vi "VideoRecorderMini.vi"() -> ()   [LabVIEW 2010]
uses:
  <instrlib>/niHWS/nihws.llb/niHWS Open File Permissions ID.ctl
  <vilib>/DAQmx/read.llb/DAQmx Read (Analog 1D Wfm NChan NSamp).vi
  <vilib>/DAQmx/create/channels.llb/DAQmx Create Channel (AI-Voltage-Basic).vi
  <vilib>/DAQmx/configure/timing.llb/DAQmx Timing (Sample Clock).vi
  <vilib>/daqmx/miscellaneous.llb/DAQmx Fill In Error Info.vi
  <instrlib>/niHWS/nihws.llb/niHWS Write Analog WDT.vi
  <instrlib>/niHWS/nihws.llb/niHWS Write Analog DBL.vi
  <vilib>/vision/driver/NI_Vision_Acquisition_Software.lvlib
  C:/Program Files/National Instruments/LabVIEW 2010/resource/objmgr/imaqdx.rc
  <vilib>/ptbypt/NI_PtbyPt.lvlib
  C:/Program Files/National Instruments/LabVIEW 2010/resource/objmgr/daqmx.rc
  <vilib>/vision/NI_Vision_Development_Module.lvlib
panel:
  in  "Ephys":bool=TRUE
  in  "Video":bool=TRUE
  in  "Downsampling factor":i32=15
  in  "reduce size":bool
  in  "Channel Names":string[](array[string])
  out "Ephys Recoding Signals":waveform(dbl)[](graph)
  in  "Recording channels":tag="PXI1Slot2/ai2"
  in  "Extra":bool=TRUE
  in  "Camera":string(combo)
  in  "Video Modes":string(combo)
  in  "Compressor":string(combo)
  in  "Selected Path for AVI":path
  in  "Rec":bool
  out "fps":dbl format="%#_2g"
  in  "% Quality":i32=-1
  in  "Start":bool
  in  "Display":bool
  out "Rec Time":dbl format="%#_3g"
  in  "stop":bool
  out "Image Out":T1(plugin-control)
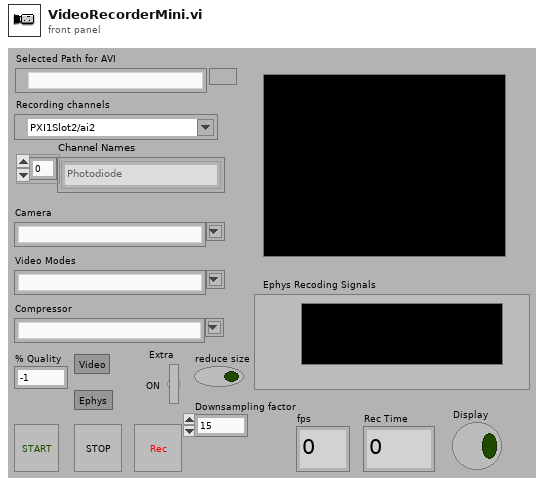
[diagram p1: front panel]
types:
  T1 = typedef "IMAQ Image.ctl" = refnum<image>
  T2 = typedef "niHWS Open File Permissions ID.ctl" = enum32{"Read Only", "Read/Write Existing", "Read/Write/Create New", "Read/Write/Create New Always"}
  T3 = cluster{"Type":u32, "Version":u32, "Flags":u32, "SerialNumberHigh":u32, "SerialNumberLow":u32, "BusType":u32, "InterfaceName":string, "VendorName":string, "ModelName":string, "CameraFileName":string, "CameraAttributeURL":string}[]
  T4 = cluster{"Type":u32, "Version":u32, "Flags":u32, "SerialNumberHigh":u32, "SerialNumberLow":u32, "BusType":u32, "InterfaceName":string, "VendorName":string, "ModelName":string, "CameraFileName":string, "CameraAttributeURL":string}
  T5 = typedef "IMAQdx.ctl" = refnum<k21>
  T6 = cluster{"Video Mode":u32, "Video Mode Name":string}[]
  T7 = typedef "AviRefnum.ctl" = refnum<k1>
  T8 = typedef "Image Type" = u32
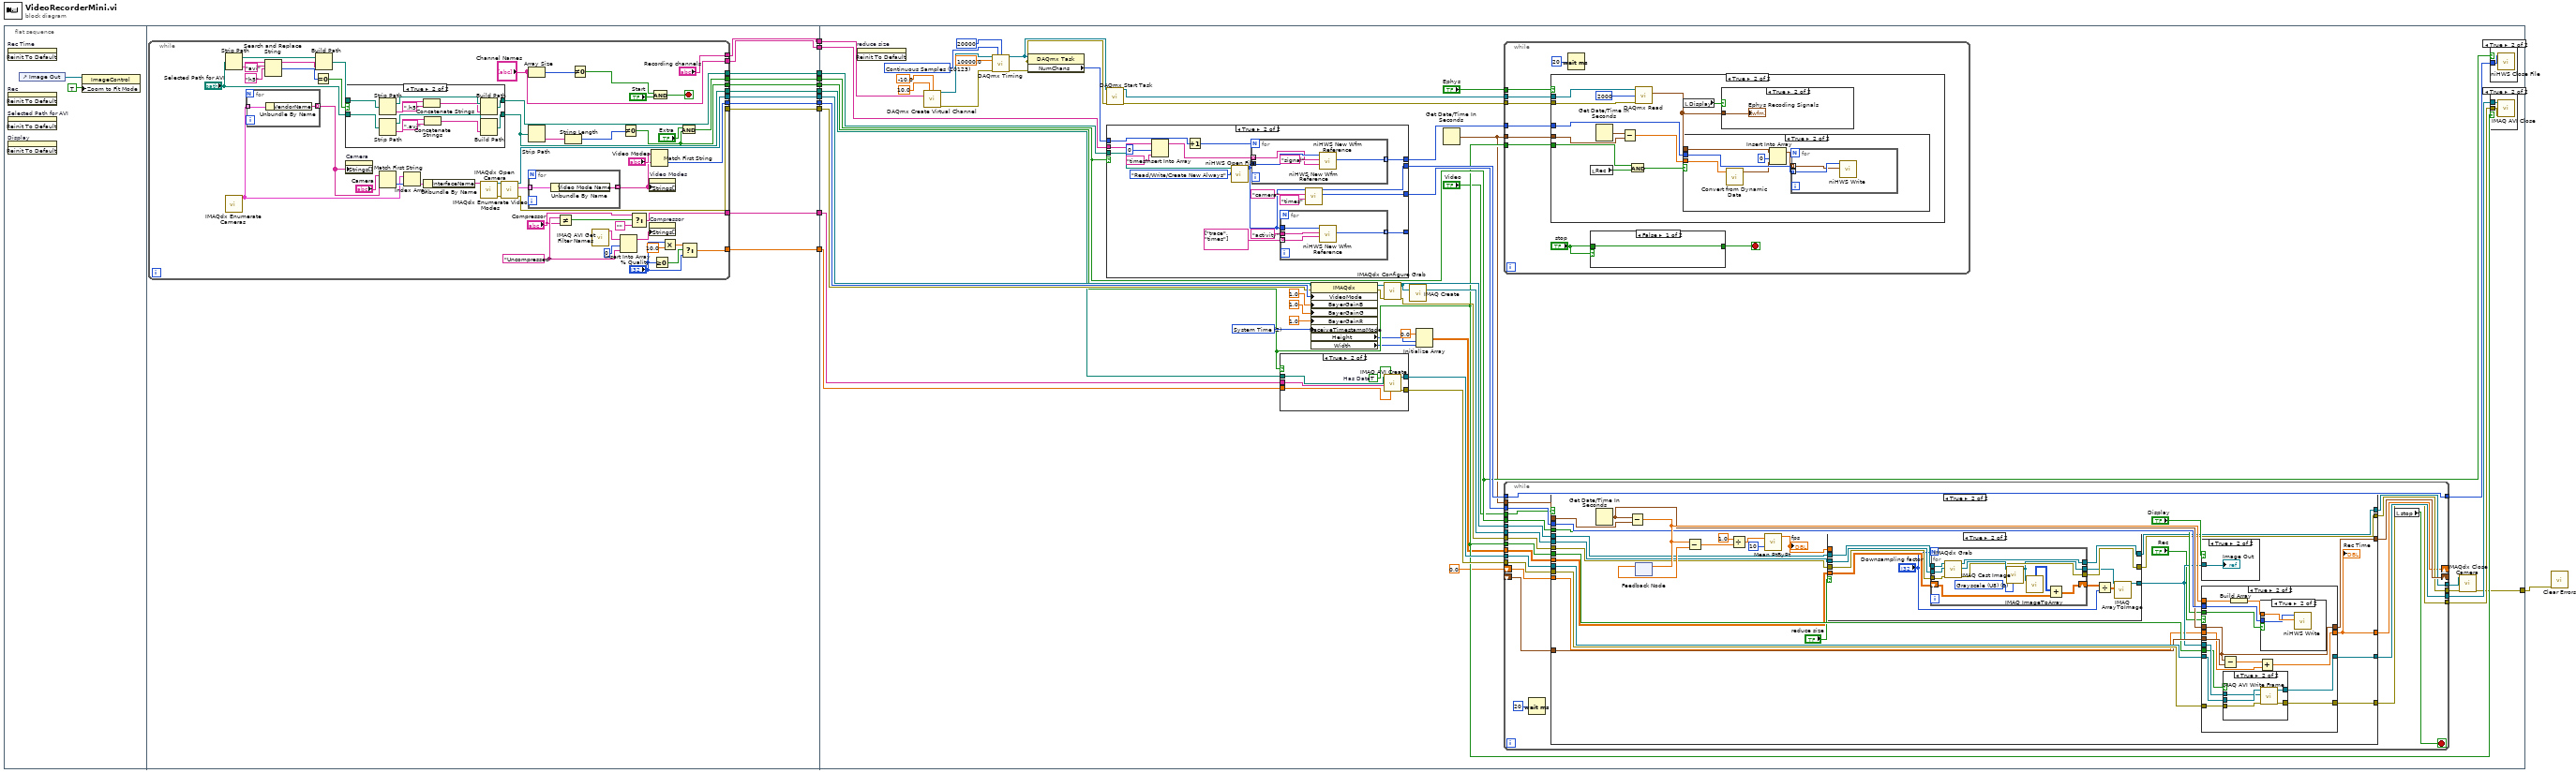
[diagram p0: block diagram]
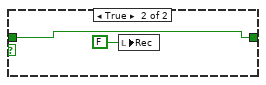
[diagram p6: hidden frame]
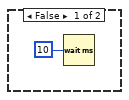
[diagram p11: hidden frame]
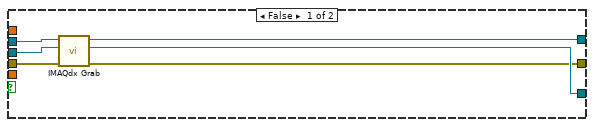
[diagram p12: hidden frame]
diagram:
  n1 = flat-sequence {
    tunnel: [w25] -> w12
    tunnel: [w24] -> w11
    tunnel: [w23] -> w10
    tunnel: [w22] -> w9
    tunnel: [w21] -> w8
    tunnel: [w20] -> w7
    tunnel: [w19] -> w6
    tunnel: [w18] -> w5
    tunnel: [w17] -> w4
    tunnel: [w16] -> w3
    tunnel: [w15] -> w2
    tunnel: w12 -> [w132]
    tunnel: w11 -> [w128]
    tunnel: w10 -> [w131]
    tunnel: w9 -> [w130]
    tunnel: w8 -> [w121]
    tunnel: w7 -> [w126]
    tunnel: w6 -> [w122]
    tunnel: w5 -> [w120]
    tunnel: w4 -> [w104]
    tunnel: w3 -> [w111]
    tunnel: w2 -> [w108]
    tunnel: [w93] -> w1
    frame #0 {
      n2 = invoke on="Rec Time" class="DigNum (strict)" method="Reinit To Default"() -> ()  [unwired: 3 in, 3 out]
      n3 = invoke on="Rec" class="Bool (strict)" method="Reinit To Default"() -> ()  [unwired: 3 in, 3 out]
      n4 = invoke on="Selected Path for AVI" class="Path" method="Reinit To Default"() -> ()  [unwired: 3 in, 3 out]
      n5 = invoke on="Display" class="Bool (strict)" method="Reinit To Default"() -> ()  [unwired: 3 in, 3 out]
      n6 = control-ref of="Image Out"() -> (w14:refnum<vi>)
      n7 = property on="Property Node" class="ImageControl"(reference=w14, "Zoom to Fit Mode"=TRUE) -> ()  [unwired: 1 in, 2 out]
    }
    frame #1 {
      n8 = while {
        tunnel: [w55] -> w25
        tunnel: [w69] -> w24
        tunnel: [w45] -> w23
        tunnel: [w62] -> w22
        tunnel: [w35] -> w21
        tunnel: [w38] -> w20
        tunnel: [w54] -> w19
        tunnel: [w32] -> w18
        tunnel: [w33] -> w17
        tunnel: ["Recording channels"] -> w16
        tunnel: ["Channel Names"] -> w15
        stop <- w26 stop-if-true
        w67 = "Uncompressed"
        n9 = Strip Path(path="Selected Path for AVI") -> (stripped path=w53:path, name=w51:string)
        n10 = call <vilib>:"IMAQdx Enumerate Cameras.vi"() -> ("Camera Information Array"=w58:T3)  [unwired: 10 in, 1 out]
        n11 = for {
          tunnel: w58 -> [w90] mode=indexing
          tunnel: [w89] -> w61 mode=indexing
          n12 = Unbundle By Name(w90) -> ("VendorName"=w89:string)
        }
        n13 = Search and Replace String(input string=w51, search string="avi", replace string="h5" ("replace string (\"\")")) -> (result string=w52:string, number of replacements=w41:i32)  [unwired: 5 in, 2 out]
        n14 = Equal To 0?(x=w41) -> (x = 0?=w40:bool)
        n15 = Build Path(base path=w53, name or relative path=w52) -> (appended path=w39:path)
        n16 = case shown="True" w40 {
          tunnel: "Selected Path for AVI" -> [w75 w88]
          tunnel: [w75 w87] -> w35
          tunnel: w39 -> [w76 w78]
          tunnel: [w76 w77] -> w38
          frame False {
          }
          frame True {
            n17 = Strip Path(path=w78) -> (stripped path=w82:path, name=w80:string)
            n18 = Strip Path(path=w88) -> (stripped path=w86:path, name=w84:string)
            n19 = Concatenate Strings(w80, ".h5" ("search string")) -> (w79:string)
            n20 = Concatenate Strings(w84, ".avi" ("search string")) -> (w83:string)
            n21 = Build Path(base path=w82, name or relative path=w79) -> (appended path=w77:path)
            n22 = Build Path(base path=w86, name or relative path=w83) -> (appended path=w87:path)
          }
        }
        n23 = property on="Camera" class="CmbBox"("Strings[]"=w61) -> ()  [unwired: 2 in, 2 out]
        n24 = Match First String(2:w61, 3:"Camera") -> (0:w59:i32)  [unwired: 1 out]
        n25 = Index Array(array=w58, index=w59) -> (element=w57:T4)
        n26 = Unbundle By Name(w57) -> ("InterfaceName"=w56:string)
        n27 = call <vilib>:"IMAQdx Open Camera.vi"("Session In"=w56) -> ("error out"=w73:errorcluster, "Session Out"=w74:T5)  [unwired: 9 in]
        n28 = call <vilib>:"IMAQdx Enumerate Video Modes.vi"("error in"=w73, "Session In"=w74) -> ("error out"=w54:errorcluster, "Video Modes"=w70:T6, "Session Out"=w55:T5)  [unwired: 6 in, 1 out]
        n29 = Array Size(array="Channel Names") -> (size(s)=w29:i32)
        n30 = Strip Path(path=w35) -> (name=w36:string)  [unwired: 1 out]
        n31 = for {
          tunnel: w70 -> [w92] mode=indexing
          tunnel: [w91] -> w63 mode=indexing
          n32 = Unbundle By Name(w92) -> ("Video Mode Name"=w91:string)
        }
        n33 = Not Equal?(x=w67, y="Compressor") -> (x != y?=w65:bool)
        n34 = String Length(string=w36) -> (length=w37:i32)
        n35 = Not Equal To 0?(x=w29) -> (x != 0?=w28:bool)
        n36 = call "IMAQ AVI Get Filter Names"() -> ("Filter Names"=w43:string[])  [unwired: 10 in, 1 out]
        n37 = Insert Into Array(array=w43, index=0 ("Index"), new element=w67) -> (w71:string[])
        n38 = Not Equal To 0?(x=w37) -> (x != 0?=w33:bool)
        n39 = Select(t="Compressor", s=w65, f="") -> (s? t:f=w69:string)
        n40 = property on="Video Modes" class="CmbBox"("Strings[]"=w63) -> ()  [unwired: 2 in, 2 out]
        n41 = property on="Compressor" class="CmbBox"("Strings[]"=w71) -> ()  [unwired: 2 in, 2 out]
        n42 = Match First String(2:w63, 3:"Video Modes") -> (0:w62:i32)  [unwired: 1 out]
        n43 = And(x=w28, y="Start") -> (x .and. y?=w26:bool)
        n44 = Greater Or Equal To 0?(x="% Quality") -> (x >= 0?=w47:bool)
        n45 = Multiply(x="% Quality", y=10.0) -> (x*y=w48:dbl)
        n46 = And(x="Extra", y=w33) -> (x .and. y?=w32:bool)
        n47 = Select(t=w48, s=w47, f="% Quality") -> (s? t:f=w45:dbl)
      }
    }
    frame #2 {
      w115 = 10123 items=["Finite Samples"=10178, "Continuous Samples"=10123, "Hardware Timed Single Point"=12522] ("sample mode")
      w127 = u32 2 items=["None", "Tick Count", "System Time"] ("ReceiveTimestampMode")
      n48 = invoke on="reduce size" class="Bool (strict)" method="Reinit To Default"() -> ()  [unwired: 3 in, 3 out]
      n49 = call-poly <vilib>:"DAQmx Create Virtual Channel.vi"("maximum value"=10.0, "minimum value"=-10.0, "physical channels"=w111) -> ("task out"=w116:refnum<k21>, "error out"=w113:errorcluster)  [unwired: 11 in]
      n50 = call-poly <vilib>:"DAQmx Timing.vi"("task/channels in"=w116, "sample mode"=w115, "samples per channel"=20000, "rate"=10000.0, "error in"=w113) -> ("task out"=w107:refnum<k21>, "error out"=w106:errorcluster)  [unwired: 9 in]
      n51 = property class="DAQmx Task"(reference=w107, error in=w106) -> ("NumChans"=w105:u32)  [unwired: 2 out]
      n52 = call <vilib>:"DAQmx Start Task.vi"("task/channels in"=w107, "error in"=w106) -> ("task out"=w110:refnum<k21>, "error out"=w109:errorcluster)  [unwired: 12 in]
      n53 = case shown="True" w120 {
        tunnel: w126 -> [_ w199]
        tunnel: [_ w198] -> w125
        tunnel: [_ w197] -> w124
        tunnel: [_ w196] -> w119
        tunnel: w108 -> [_ w195]
        tunnel: w105 -> [_ w191]
        tunnel: [_ w188] -> _
        frame False {
        }
        frame True {
          n54 = Insert Into Array(array=w195, index=0, new element="times" ("group name (empty)")) -> (w192:string[])
          n55 = Increment(x=w191) -> (x+1=w190:u32)
          n56 = call <instrlib>:"niHWS Open File.vi"("permissions (0:read only)"=niHWS_Open_File_Permissions_ID."Read/Write/Create New Always", "file path"=w199) -> ("file handle"=w189:u32)  [unwired: 8 in, 1 out]
          n57 = for {
            N: w190 -> [_]
            tunnel: w189 -> [w209]
            tunnel: [w208] -> w196 mode=indexing
            tunnel: w192 -> [w207] mode=indexing
            n58 = call <instrlib>:"niHWS New Wfm Reference.vi"("waveform name (empty)"=w207, "group name (empty)"="signal", "file handle in"=w209) -> ("waveform reference"=w208:u32)  [unwired: 6 in, 2 out]
          }
          n59 = for {
            tunnel: w189 -> [w206]
            tunnel: [w205] -> w188 mode=indexing
            tunnel: "activity" ("group name (empty)") -> [w204]
            tunnel: string[] ["trace", "times"] -> [w203] mode=indexing
            n60 = call <instrlib>:"niHWS New Wfm Reference.vi"("waveform name (empty)"=w203, "group name (empty)"=w204, "file handle in"=w206) -> ("waveform reference"=w205:u32)  [unwired: 6 in, 2 out]
          }
          n61 = call <instrlib>:"niHWS New Wfm Reference.vi"("waveform name (empty)"="times" ("group name (empty)"), "group name (empty)"="camera", "file handle in"=w189) -> ("waveform reference"=w198:u32, "file handle out"=w197:u32)  [unwired: 6 in, 1 out]
        }
      }
      n62 = case shown="True" w104 {
        tunnel: [_ w183] -> w143
        tunnel: [_ w182] -> w140
        tunnel: w131 -> [_ w181]
        tunnel: w128 -> [_ w180]
        tunnel: w121 -> [_ w179]
        frame False {
        }
        frame True {
          w184 = TRUE  # Has Data
          n63 = call "IMAQ AVI Create"("quality"=w181, "Has Data"=w184, "Compression Filter"=w180, "AVI Path"=w179) -> ("error out"=w182:errorcluster, "Avi Refnum"=w183:T7)  [unwired: 3 in, 3 out]
        }
      }
      n64 = property class="IMAQdx"(reference=w132, error in=w122, "VideoMode"=w130, "BayerGainB"=1.0, "BayerGainG"=1.0, "BayerGainR"=1.0, "ReceiveTimestampMode"=w127) -> (reference out=w134:T5, error out=w133:errorcluster, "Height"=w102:u32, "Width"=w101:u32)
      n65 = call <vilib>:"IMAQdx Configure Grab.vi"("error in"=w133, "Session In"=w134) -> ("error out"=w138:errorcluster, "Session Out"=w129:T5)  [unwired: 8 in]
      n66 = call "IMAQ Create"("Image Name"=w129) -> ("New Image"=w139:T1)  [unwired: 4 in, 1 out]
      n67 = Initialize Array(0.0 ("element"), w102, w101) -> (w100:dbl[][])
      n68 = Get Date/Time In Seconds() -> (seconds since 1Jan1904=w96:timestamp)
      n69 = while {
        tunnel: w119 -> [w152]
        tunnel: w110 -> [w151]
        tunnel: w109 -> [w150]
        tunnel: w96 -> [w149]
        tunnel: w104 -> [w147]
        tunnel: "Ephys" -> [w144]
        stop <- w145 stop-if-true
        n70 = case shown="True" w144 {
          tunnel: w152 -> [_ w164]
          tunnel: w151 -> [_ w162]
          tunnel: w150 -> [_ w161]
          tunnel: w149 -> [_ w158]
          tunnel: w147 -> [_ w155]
          frame False {
          }
          frame True {
            n71 = local read "Rec"() -> (w154:bool)
            n72 = Get Date/Time In Seconds() -> (seconds since 1Jan1904=w159:timestamp)
            n73 = Subtract(x=w159, y=w158) -> (x-y=w157:dbl)
            n74 = And(x=w155, y=w154) -> (x .and. y?=w153:bool)
            n75 = call-poly <vilib>:"DAQmx Read.vi"("task/channels in"=w162, "number of samples per channel"=2000, "error in"=w161) -> ("data"=w160:waveform(dbl)[])  [unwired: 10 in, 2 out]
            n76 = local read "Display"() -> (w156:bool)
            n77 = case shown="True" w153 {
              tunnel: w164 -> [_ w171]
              tunnel: w160 -> [_ w169]
              tunnel: w157 -> [_ w170]
              frame False {
              }
              frame True {
                n78 = call "Convert from Dynamic Data"("Dynamic Data Type"=w170) -> ("Waveform"=w168:waveform(dbl))  [unwired: 3 in]
                n79 = Insert Into Array(array=w169, index=0, new element=w168) -> (w166:waveform(dbl)[])
                n80 = for {
                  tunnel: w171 -> [w173] mode=indexing
                  tunnel: w166 -> [w172] mode=indexing
                  n81 = call-poly <instrlib>:"niHWS Write.vi"("analog waveform"=w172, "waveform reference in"=w173) -> ()  [unwired: 8 in, 2 out]
                }
              }
            }
            n82 = case shown="True" w156 {
              tunnel: w160 -> [_ w165]
              frame False {
              }
              frame True {
                "Ephys Recoding Signals" <- w165
              }
            }
          }
        }
        n83 = Wait (ms)(milliseconds to wait=u32 20) -> ()  [unwired: 1 out]
        n84 = case shown="False" "stop" {
          tunnel: "stop" -> [w174 w175]
          tunnel: [w174 w175] -> w145
          frame False {
          }
          frame True {
            n85 = local write "Rec"(FALSE ("Rec")) -> ()
          }
        }
      }
      n86 = while {
        tunnel: [w232] -> w142
        tunnel: [w231] -> w141
        tunnel: w143 -> [w230]
        tunnel: w140 -> [w229]
        tunnel: w139 -> [w219]
        tunnel: w129 -> [w220]
        tunnel: w138 -> [w218]
        tunnel: w96 -> [w228]
        tunnel: w125 -> [w227]
        tunnel: w124 -> [w226]
        tunnel: [w226] -> w123
        shift-right: [w225] -> _
        shift-left: _ -> [w224]
        tunnel: w120 -> [w222]
        tunnel: w104 -> [w223]
        tunnel: w100 -> [w221]
        tunnel: [w217] -> w99
        tunnel: [w216] -> w98
        shift-right: [w214] -> _
        shift-left: 0.0 -> [w215]
        tunnel: "Video" -> [w213]
        stop <- w212 stop-if-true
        n87 = Wait (ms)(milliseconds to wait=u32 20) -> ()  [unwired: 1 out]
        n88 = case shown="True" w213 {
          tunnel: [_ w263] -> w232
          tunnel: [_ w262] -> w231
          tunnel: w230 -> [_ w261]
          tunnel: w229 -> [_ w260]
          tunnel: w228 -> [_ w258]
          tunnel: w227 -> [_ w252]
          tunnel: [_ w250] -> w225
          tunnel: w224 -> [_ w249]
          tunnel: w223 -> [_ w247]
          tunnel: w222 -> [_ w246]
          tunnel: w221 -> [_ w243]
          tunnel: w220 -> [_ w242]
          tunnel: w219 -> [_ w241]
          tunnel: w218 -> [_ w240]
          tunnel: [_ w239] -> w217
          tunnel: [_ w238] -> w216
          tunnel: w215 -> [_ w237]
          tunnel: [_ w236] -> w214
          frame False {
            n89 = Wait (ms)(milliseconds to wait=u32 10) -> ()  [unwired: 1 out]
          }
          frame True {
            n90 = Get Date/Time In Seconds() -> (seconds since 1Jan1904=w251:timestamp)
            n91 = Subtract(x=w251, y=w258) -> (x-y=w253:dbl)
            n92 = feedback #1() -> (w257:dbl)  [unwired: 1 in]
            n93 = feedback-in #1(w253) -> ()
            n94 = Subtract(x=w253, y=w257) -> (x-y=w255:dbl)
            n95 = Divide(x=1.0, y=w255) -> (x/y=w254:dbl)
            n96 = call <vilib>:"Mean PtByPt.vi"("x"=w254, "sample length"=10) -> ("mean"=w235:dbl)  [unwired: 2 in, 1 out]
            "fps" <- w235
            n97 = case shown="True" "reduce size" {
              tunnel: [w269 w274] -> w245
              tunnel: w235 -> [_ _]
              tunnel: w243 -> [_ w280]
              tunnel: w242 -> [w268 w279]
              tunnel: w241 -> [w267 w278]
              tunnel: w240 -> [w266 w277]
              tunnel: [w264 w276] -> w238
              tunnel: [w265 w275] -> w239
              frame False {
                n98 = call <vilib>:"IMAQdx Grab.vi"("error in"=w266, "Image In"=w267, "Session In"=w268) -> ("error out"=w264:errorcluster, "Image Out"=w269:T1, "Session Out"=w265:T5)  [unwired: 5 in, 1 out]
              }
              frame True {
                n99 = for {
                  N: "Downsampling factor" -> [_]
                  tunnel: w279 -> [w291]
                  tunnel: w278 -> [w290]
                  tunnel: w277 -> [w288]
                  tunnel: [w287] -> w276
                  tunnel: [w286] -> w275
                  shift-right: [w282] -> w273
                  shift-left: w280 -> [w283]
                  tunnel: [w281] -> w271
                  w285 = T8 0 items=["Grayscale (U8)", "Grayscale (I16)", "Grayscale (SGL)", "Complex (CSG)", "RGB (U32)", "HSL (U32)", "RGB (U64)", "Grayscale (U16)"] ("Image Type")
                  n100 = call <vilib>:"IMAQdx Grab.vi"("error in"=w288, "Image In"=w290, "Session In"=w291) -> ("error out"=w287:errorcluster, "Image Out"=w289:T1, "Session Out"=w286:T5)  [unwired: 5 in, 1 out]
                  n101 = call "IMAQ Cast Image"("Image Type"=w285, "Image Src"=w289) -> ("Image Dst Out"=w281:T1)  [unwired: 8 in, 1 out]
                  n102 = call "IMAQ ImageToArray"("Image"=w281) -> ("Image Pixels (U8)"=w284:u8[][])  [unwired: 3 in, 4 out]
                  n103 = Add(x=w284, y=w283) -> (x+y=w282:dbl[][])
                }
                n104 = Divide(x=w273, y="Downsampling factor") -> (x/y=w272:dbl[][])
                n105 = call "IMAQ ArrayToImage"("Image Pixels (U8)"=w272, "Image"=w271) -> ("Image Out"=w274:T1)  [unwired: 8 in, 1 out]
              }
            }
            n106 = case shown="True" "Display" {
              tunnel: w245 -> [_ w318]
              frame False {
              }
              frame True {
                "Image Out" <- w318
              }
            }
            n107 = case shown="True" "Rec" {
              tunnel: [w294 w310] -> w263
              tunnel: [w295 w309] -> w262
              tunnel: w261 -> [w294 w308]
              tunnel: w260 -> [w295 w307]
              tunnel: w245 -> [_ w306]
              tunnel: [w292 w296] -> w236
              tunnel: w253 -> [_ w305]
              tunnel: w252 -> [_ w303]
              tunnel: [w293 w301] -> w250
              tunnel: w251 -> [w293 w301]
              tunnel: w249 -> [_ w300]
              tunnel: w246 -> [_ w299]
              tunnel: w247 -> [_ w298]
              tunnel: w237 -> [w292 w297]
              frame False {
              }
              frame True {
                n108 = Subtract(x=w301, y=w300) -> (x-y=w302:dbl)
                n109 = case shown="True" w298 {
                  tunnel: [_ w315] -> w310
                  tunnel: [_ w314] -> w309
                  tunnel: w308 -> [_ w313]
                  tunnel: w307 -> [_ w312]
                  tunnel: w306 -> [_ w311]
                  frame False {
                  }
                  frame True {
                    n110 = call "IMAQ AVI Write Frame"("error in (no error)"=w312, "Image"=w311, "Avi Refnum"=w313) -> ("error out"=w314:errorcluster, "Avi Refnum (duplicate)"=w315:T7)  [unwired: 7 in]
                  }
                }
                n111 = Build Array(w305) -> (w304:dbl[])
                n112 = Add(x=w302, y=w297) -> (x+y=w296:dbl)
                n113 = case shown="True" w299 {
                  tunnel: w304 -> [_ w317]
                  tunnel: w303 -> [_ w316]
                  frame False {
                  }
                  frame True {
                    n114 = call-poly <instrlib>:"niHWS Write.vi"("data"=w317, "waveform reference in"=w316) -> ()  [unwired: 8 in, 2 out]
                  }
                }
              }
            }
            "Rec Time" <- w236
          }
        }
        n115 = local read "stop"() -> (w212:bool)
      }
      n116 = call <vilib>:"IMAQdx Close Camera.vi"("error in"=w98, "Session In"=w99) -> ("error out"=w93:errorcluster)  [unwired: 9 in]
      n117 = case shown="True" w120 {
        tunnel: w123 -> [_ w185]
        frame False {
        }
        frame True {
          n118 = call <instrlib>:"niHWS Close File.vi"("file handle"=w185) -> ()  [unwired: 10 in, 1 out]
        }
      }
      n119 = case shown="True" w104 {
        tunnel: w142 -> [_ w178]
        tunnel: w141 -> [_ w177]
        frame False {
        }
        frame True {
          n120 = call "IMAQ AVI Close"("error in (no error)"=w177, "Avi Refnum"=w178) -> ()  [unwired: 9 in, 1 out]
        }
      }
    }
  }
  n121 = call <vilib>:"Clear Errors.vi"("error in (no error)"=w1) -> ()  [unwired: 6 in, 1 out]
